vi "Taskbar Progress bar Example.vi"   [LabVIEW 2010]
doc: "This example shows how to use the LabVIEW Taskbar Progress Bar API."
uses:
  _TypeDefs/Progress State.ctl
  TaskbarProgressAPI.lvlib
panel:
  # "Run this VI and watch the show on the LabVIEW Taskbar button!"
types:
  T1 = typedef "TaskbarProgressAPI.lvlib/Progress State.ctl" = i32
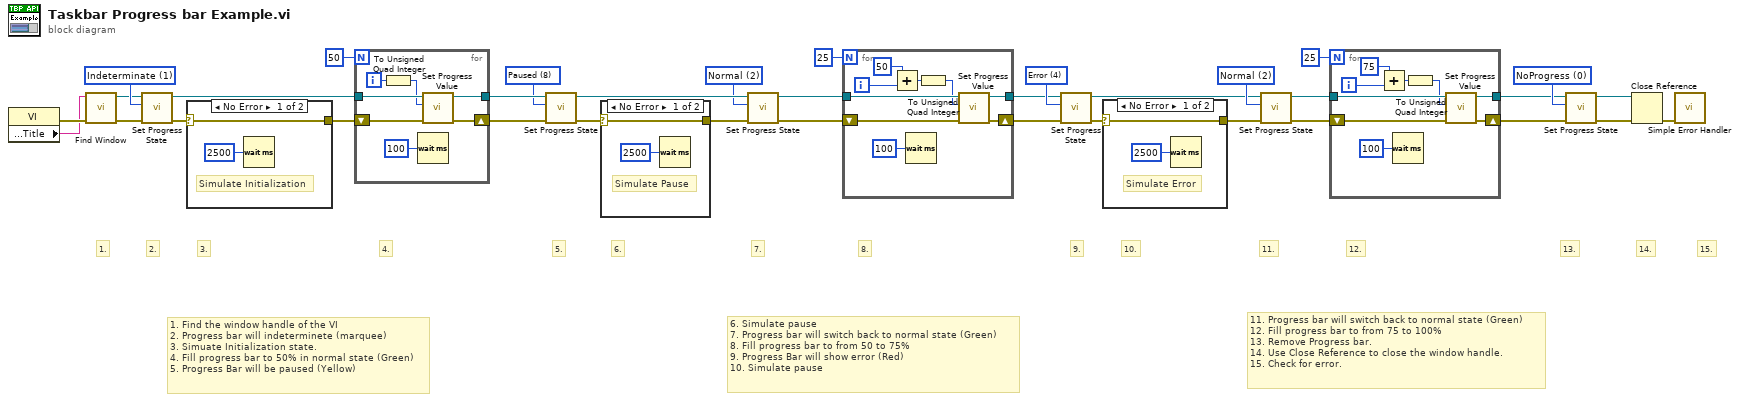
[diagram p0: block diagram]
diagram:
  w13 = T1 2 items=["NoProgress"=0, "Indeterminate"=1, "Normal"=2, "Error"=4, "Paused"=8] ("State (No Progress)")
  w16 = T1 4 items=["NoProgress"=0, "Indeterminate"=1, "Normal"=2, "Error"=4, "Paused"=8] ("State (No Progress)")
  w17 = T1 2 items=["NoProgress"=0, "Indeterminate"=1, "Normal"=2, "Error"=4, "Paused"=8] ("State (No Progress)")
  w22 = T1 0 items=["NoProgress"=0, "Indeterminate"=1, "Normal"=2, "Error"=4, "Paused"=8] ("State (No Progress)")
  w24 = T1 8 items=["NoProgress"=0, "Indeterminate"=1, "Normal"=2, "Error"=4, "Paused"=8] ("State (No Progress)")
  w31 = T1 1 items=["NoProgress"=0, "Indeterminate"=1, "Normal"=2, "Error"=4, "Paused"=8] ("state")
  # "11. Progress bar will switch back to normal state (Green)\n12. Fill progress bar to from 75 to 100%\n13. Remove Progress bar.\n14. Use Close Reference to close the window handle.\n15. Check for error."
  # "15."
  # "14."
  # "13."
  # "12."
  # "11."
  # "10."
  # "9."
  # "8."
  # "6. Simulate pause\n7. Progress bar will switch back to normal state (Green)\n8. Fill progress bar to from 50 to 75% \n9. Progress Bar will show error (Red)\n10. Simulate pause"
  # "1. Find the window handle of the VI\n2. Progress bar will indeterminete (marquee)\n3. Simuate Initialization state.\n4. Fill progress bar to 50% in normal state (Green)\n5. Progress Bar will be paused (Yellow)"
  # "7."
  # "6."
  # "5."
  # "4."
  # "3."
  # "2."
  # "1."
  n1 = property class="VI"() -> (error out=w34:errorcluster, "Front Panel.Title"=w33:string)  [unwired: 2 in, 1 out]
  n2 = call "Find Window.vi"("error in (no error)"=w34, "Window Title (Callers Window)"=w33) -> ("error out"=w32:errorcluster, "Window Handle"=w30:refnum<k24>)  [unwired: 8 in]
  n3 = call "Set Progress State.vi"("error in (no error)"=w32, "State (No Progress)"=w31, "Window Handle"=w30) -> ("error out"=w6:errorcluster, "dup Window Handle"=w29:refnum<k24>)  [unwired: 7 in]
  n4 = case shown="No Error" w6 {
    selector: w6 -> [w36 w38]
    tunnel: [w36 w38] -> w5
    frame No Error {
      # "Simulate Initialization"
      n5 = Wait (ms)(milliseconds to wait=u32 2500) -> ()  [unwired: 1 out]
    }
    frame Error {
    }
  }
  n6 = for {
    N: 50 -> [_]
    tunnel: w29 -> [w44]
    shift-right: [w41] -> w26
    shift-left: w5 -> [w45]
    tunnel: [w39] -> w27
    i -> [w43]
    n7 = To Unsigned Quad Integer(1:w43) -> (0:w42:u64)
    n8 = Wait (ms)(milliseconds to wait=u32 100) -> ()  [unwired: 1 out]
    n9 = call "Set Progress Value.vi"("error in (no error)"=w45, "current (0)"=w42, "Window Handle"=w44) -> ("error out"=w41:errorcluster, "dup Window Handle"=w39:refnum<k24>)  [unwired: 7 in]
  }
  n10 = call "Set Progress State.vi"("error in (no error)"=w26, "State (No Progress)"=w24, "Window Handle"=w27) -> ("error out"=w4:errorcluster, "dup Window Handle"=w18:refnum<k24>)  [unwired: 7 in]
  n11 = case shown="No Error" w4 {
    selector: w4 -> [w46 w48]
    tunnel: [w46 w48] -> w3
    frame No Error {
      # "Simulate Pause"
      n12 = Wait (ms)(milliseconds to wait=u32 2500) -> ()  [unwired: 1 out]
    }
    frame Error {
    }
  }
  n13 = call "Set Progress State.vi"("error in (no error)"=w3, "State (No Progress)"=w17, "Window Handle"=w18) -> ("error out"=w20:errorcluster, "dup Window Handle"=w19:refnum<k24>)  [unwired: 7 in]
  n14 = for {
    N: 25 -> [_]
    tunnel: w19 -> [w56]
    shift-right: [w55] -> w14
    shift-left: w20 -> [w57]
    tunnel: [w53] -> w15
    i -> [w52]
    n15 = Add(x=50, y=w52) -> (x+y=w50:i32)
    n16 = Wait (ms)(milliseconds to wait=u32 100) -> ()  [unwired: 1 out]
    n17 = To Unsigned Quad Integer(1:w50) -> (0:w49:u64)
    n18 = call "Set Progress Value.vi"("error in (no error)"=w57, "current (0)"=w49, "Window Handle"=w56) -> ("error out"=w55:errorcluster, "dup Window Handle"=w53:refnum<k24>)  [unwired: 7 in]
  }
  n19 = call "Set Progress State.vi"("error in (no error)"=w14, "State (No Progress)"=w16, "Window Handle"=w15) -> ("error out"=w2:errorcluster, "dup Window Handle"=w12:refnum<k24>)  [unwired: 7 in]
  n20 = case shown="No Error" w2 {
    selector: w2 -> [w58 w60]
    tunnel: [w58 w60] -> w1
    frame No Error {
      # "Simulate Error"
      n21 = Wait (ms)(milliseconds to wait=u32 2500) -> ()  [unwired: 1 out]
    }
    frame Error {
    }
  }
  n22 = call "Set Progress State.vi"("error in (no error)"=w1, "State (No Progress)"=w13, "Window Handle"=w12) -> ("error out"=w9:errorcluster, "dup Window Handle"=w10:refnum<k24>)  [unwired: 7 in]
  n23 = for {
    N: 25 -> [_]
    tunnel: w10 -> [w68]
    shift-right: [w67] -> w8
    shift-left: w9 -> [w69]
    tunnel: [w65] -> w7
    i -> [w64]
    n24 = Add(x=75, y=w64) -> (x+y=w62:i32)
    n25 = Wait (ms)(milliseconds to wait=u32 100) -> ()  [unwired: 1 out]
    n26 = To Unsigned Quad Integer(1:w62) -> (0:w61:u64)
    n27 = call "Set Progress Value.vi"("error in (no error)"=w69, "current (0)"=w61, "Window Handle"=w68) -> ("error out"=w67:errorcluster, "dup Window Handle"=w65:refnum<k24>)  [unwired: 7 in]
  }
  n28 = call "Set Progress State.vi"("error in (no error)"=w8, "State (No Progress)"=w22, "Window Handle"=w7) -> ("error out"=w23:errorcluster, "dup Window Handle"=w21:refnum<k24>)  [unwired: 7 in]
  n29 = Close Reference(reference=w21, error in (no error)=w23) -> (error out=w35:errorcluster)
  n30 = call <vilib>:"Simple Error Handler.vi"("error in (no error)"=w35) -> ()  [unwired: 4 in, 5 out]
